vi "SysDef.CreateDescription.vi"(8 "error in (no error)":errorcluster, 10 "Description":string, 11 "ID in":T1 format="%.0x") -> (0 "error out":errorcluster, 3 "ID out":T1 format="%.0x")   [LabVIEW 2015, in "Import - Export CD Config Utility.lvlib"]
uses:
  Import - Export CD Config Utility.lvlib
  <vilib>/NI Veristand/Custom Device API/Custom Device Item Ref.ctl
  NationalInstruments.VeriStand.SystemDefinitionAPI
  <vilib>/NI Veristand/Custom Device API/Custom Device API.lvlib
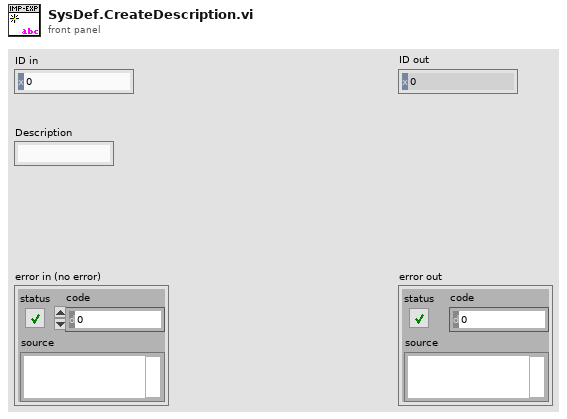
[diagram p1: front panel]
types:
  T1 = typedef "Custom Device API.lvlib/Custom Device Item Ref.ctl" = u64
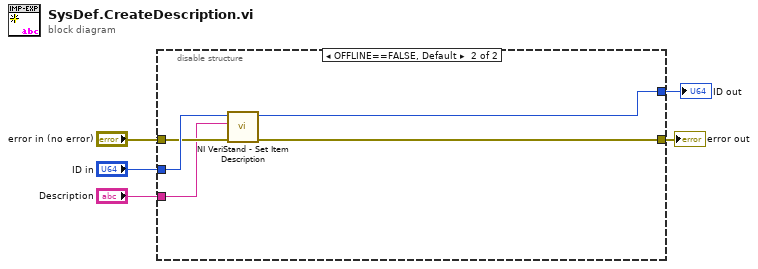
[diagram p0: block diagram]
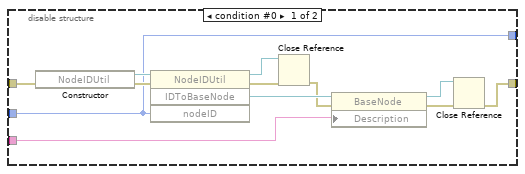
[diagram p2: hidden frame]
diagram:
  n1 = disable-structure shown="OFFLINE==FALSE, Default" {
    disable-tunnel: "ID in" -> [w6 w22]
    disable-tunnel: "Description" -> [w9 w20]
    disable-tunnel: "error in (no error)" -> [w8 w21]
    disable-tunnel: [w7 w19] -> w2
    disable-tunnel: [w6 w18] -> w1
    frame condition #0 {
      n2 = constructor class="NodeIDUtil"(error in=w8) -> (reference out=w17:refnum<k24>, error out=w16:errorcluster)  [unwired: 2 in, 1 out]
      n3 = invoke class="NodeIDUtil" method="IDToBaseNode"(reference=w17, error in=w16, "nodeID"=w6) -> (reference out=w14:refnum<k24>, error out=w15:errorcluster, "IDToBaseNode"=w11:refnum<k24>)  [unwired: 1 in, 1 out]
      n4 = Close Reference(reference=w14, error in (no error)=w15) -> (error out=w10:errorcluster)
      n5 = property class="BaseNode"(reference=w11, error in=w10, "Description"=w9) -> (reference out=w13:refnum<k24>, error out=w12:errorcluster)
      n6 = Close Reference(reference=w13, error in (no error)=w12) -> (error out=w7:errorcluster)
    }
    frame condition #1 (active) {
      n7 = call <vilib>:"NI VeriStand - Set Item Description.vi"("error in (no error)"=w21, "Description"=w20, "Item Ref in"=w22) -> ("error out"=w19:errorcluster, "Item Ref out"=w18:T1)  [unwired: 6 in, 1 out]
    }
  }
  "error out" <- w2
  "ID out" <- w1
